vi "Read from RAM.vi"(8 "error in (no error)":errorcluster, 9 "size":u16, 10 "address":u16, 11 "TroSpec in":refnum<class "PL ISTEQ TroSpec.lvclass">) -> (0 "error out":errorcluster, 2 "data":u8[](array[numeric]), 3 "TroSpec out":refnum<class "PL ISTEQ TroSpec.lvclass">)   [LabVIEW 2015, in "PL ISTEQ TroSpec.lvclass"]
doc: "Reads data from RAM."
uses:
  PL ISTEQ TroSpec.lvclass
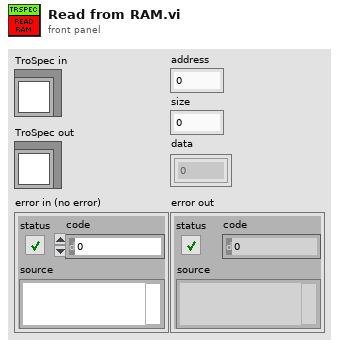
[diagram p1: front panel]
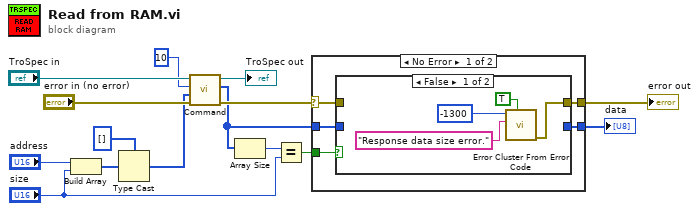
[diagram p0: block diagram]
diagram:
  n1 = Build Array("address", "size") -> (w11:u16[])
  n2 = Type Cast(type=u8[] [] ("command payload"), x=w11) -> (*(type *) &x=w9:u8[])
  n3 = call "Command.vi"("error in (no error)"="error in (no error)", "command payload"=w9, "command"=u8 10, "TroSpec in"="TroSpec in") -> ("error out"=w7:errorcluster, "response payload"=w5:u8[], "TroSpec out"=→"TroSpec out":refnum<class "PL ISTEQ TroSpec.lvclass">)  [unwired: 5 in]
  n4 = Array Size(array=w5) -> (size(s)=w4:i32)
  n5 = Equal?(x=w4, y="size") -> (x = y?=w2:bool)
  n6 = case shown="No Error" w7 {
    selector: w7 -> [w17 w27]
    tunnel: [w16 w27] -> w6
    tunnel: w5 -> [w19 _]
    tunnel: w2 -> [w20 _]
    tunnel: [w18 _] -> w1
    frame No Error {
      n7 = case shown="False" w20 {
        tunnel: w19 -> [_ w26]
        tunnel: [_ w26] -> w18
        tunnel: w17 -> [_ w25]
        tunnel: [w21 w25] -> w16
        frame False {
          n8 = call <vilib>:"Error Cluster From Error Code.vi"("show call chain? (False)"=TRUE, "error message (\"\")"="Response data size error." ("format string"), "error code (0)"=-1300) -> ("error out"=w21:errorcluster)  [unwired: 6 in]
        }
        frame True {
        }
      }
    }
    frame Error {
    }
  }
  "error out" <- w6
  "data" <- w1
